vi "BRAM Ping Pong Control Logic.vi"(8 "Input Valid":bool, 10 "Read Count":u16, 11 "Write Count":u16) -> (0 "Read Valid":bool, 2 "BRAM Bank0 Write?":bool, 3 "Read Address":u16)   [LabVIEW 2012]
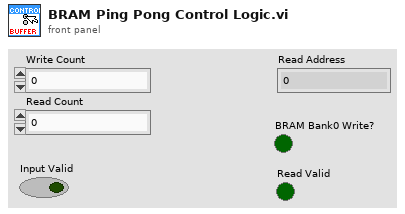
[diagram p1: front panel]
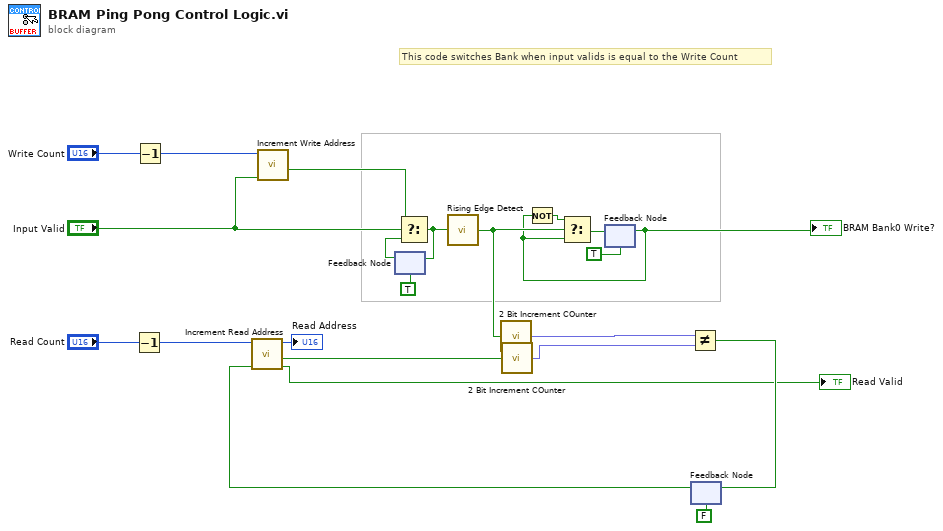
[diagram p0: block diagram]
diagram:
  # "This code switches Bank when input valids is equal to the Write Count"
  n1 = Decrement(x="Read Count") -> (x-1=w3:u16)
  n2 = Decrement(x="Write Count") -> (x-1=w4:u16)
  n3 = call <userlib>:"Increment Write Address.vi"("INC?"="Input Valid", "rollover"=w4) -> ("roll over"=w16:bool)  [unwired: 7 in, 2 out]
  n4 = feedback #1(TRUE ("roll over")) -> (w15:bool)
  n5 = Select(t=w16, s="Input Valid", f=w15) -> (s? t:f=w14:bool)
  n6 = feedback-in #1(w14) -> ()
  n7 = call <userlib>:"Rising Edge Detect.vi"("signal"=w14) -> ("edge detected"=w17:bool)  [unwired: 14 in]
  n8 = call <userlib>:"2 Bit Increment COunter.vi"("Increment"=w17) -> ("Counter Value"=w21:fxp<+,2,2>)  [unwired: 14 in]
  n9 = feedback #2(TRUE) -> (w7:bool)
  "BRAM Bank0 Write?" <- w7
  n10 = Not(x=w7) -> (.not. x?=w18:bool)
  n11 = Select(t=w18, s=w17, f=w7) -> (s? t:f=w12:bool)
  n12 = feedback-in #2(w12) -> ()
  n13 = feedback #3(FALSE) -> (w10:bool)
  n14 = call <userlib>:"Increment Read Address.vi"("INC?"=w10, "rollover"=w3) -> ("Output Valid"=→"Read Valid":bool, "roll over"=w22:bool, "count"=→"Read Address":u16)  [unwired: 7 in]
  n15 = call <userlib>:"2 Bit Increment COunter.vi"("Increment"=w22) -> ("Counter Value"=w19:fxp<+,2,2>)  [unwired: 14 in]
  n16 = Not Equal?(x=w21, y=w19) -> (x != y?=w9:bool)
  n17 = feedback-in #3(w9) -> ()
